vi "Set multiple channels.vi"(6 "timeout (ms)":i32, 8 "values":dbl[](array[numeric]), 9 "names":string[](array[string]), 10 "Gateway IP Address (\"\": localhost)":string, 11 "Sequence Context":refnum<k7>) -> (0 "error out":errorcluster, 1 "timed out?":bool, 2 "Report Text":string)   [LabVIEW 2014, in "Set Channels.lvlib"]
uses:
  Set Channels.lvlib
  <vilib>/NI Veristand/Execution/Workspace/NI VeriStand - Set Multiple Channel Values.vi
  <vilib>/NI Veristand/Execution/Workspace/NI VeriStand - Get Multiple Channel Values.vi
  <vilib>/NI Veristand/Execution/Workspace/NI_VS Workspace ExecutionAPI.lvlib
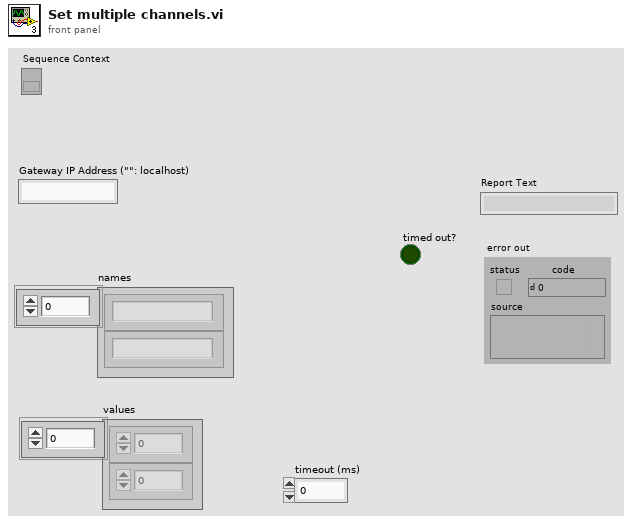
[diagram p1: front panel]
types:
  T1 = typedef "NI_VS Workspace ExecutionAPI.lvlib/WorkspaceAPI.ctl" = refnum<k24>
  T2 = typedef "TestStand - Status Monitor.ctl" = cluster{"Sequence Context":refnum<k7>, "Execution":refnum<k7>, "Termination Monitor":refnum<k7>}
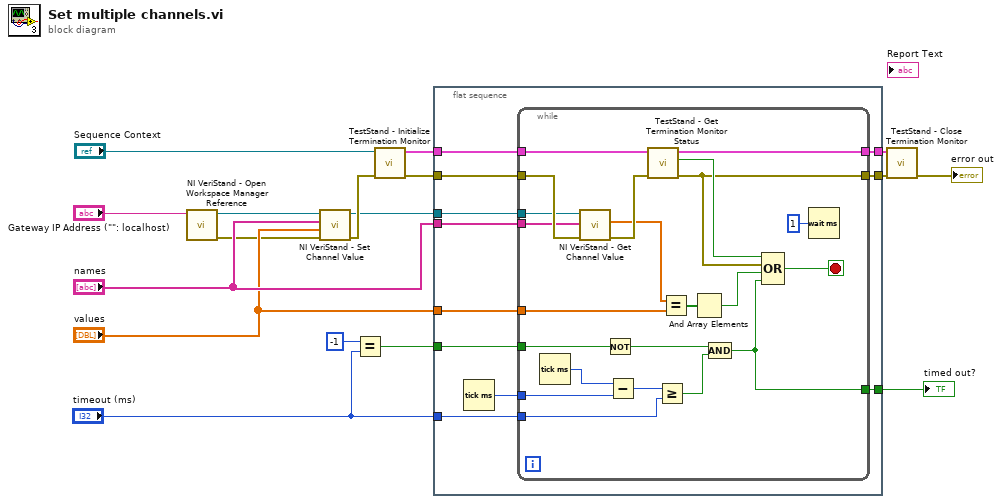
[diagram p0: block diagram]
diagram:
  n1 = call <vilib>:"NI VeriStand - Open Workspace Manager Reference.vi"("Gateway IP Address (\"\": localhost)"="Gateway IP Address (\"\": localhost)") -> ("error out"=w6:errorcluster, "WorkspaceManager"=w7:T1)  [unwired: 9 in]
  n2 = call-poly <vilib>:"NI VeriStand - Set Channel Value.vi"("error in (no error)"=w6, "Values"="values", "Channels"="names", "WorkspaceManager in"=w7) -> ("error out"=w17:errorcluster, "WorkspaceManager out"=w10:T1)  [unwired: 6 in]
  n3 = Equal?(x=-1, y="timeout (ms)") -> (x = y?=w3:bool)
  n4 = call <vilib>:"TestStand - Initialize Termination Monitor.vi"("error in (no error)"=w17, "Sequence Context In"="Sequence Context") -> ("error out"=w11:errorcluster, "Status Monitor Out"=w14:T2)  [unwired: 8 in]
  n5 = flat-sequence {
    tunnel: w14 -> [w28]
    tunnel: [w27] -> w13
    tunnel: [w26] -> w12
    tunnel: w11 -> [w25]
    tunnel: w10 -> [w24]
    tunnel: "names" -> [w23]
    tunnel: "values" -> [w22]
    tunnel: w3 -> [w20]
    tunnel: "timeout (ms)" -> [w19]
    tunnel: [w18] -> w1
    frame #0 {
      n6 = Tick Count (ms)() -> (millisecond timer value=w21:u32)
      n7 = while {
        tunnel: w28 -> [w46]
        tunnel: [w45] -> w27
        tunnel: [w44] -> w26
        tunnel: w25 -> [w42]
        tunnel: w24 -> [w41]
        tunnel: w23 -> [w40]
        tunnel: w22 -> [w39]
        tunnel: w21 -> [w36]
        tunnel: w20 -> [w30]
        tunnel: w19 -> [w32]
        tunnel: [w31] -> w18
        stop <- w43 stop-if-true
        n8 = Tick Count (ms)() -> (millisecond timer value=w35:u32)
        n9 = call-poly <vilib>:"NI VeriStand - Get Channel Value.vi"("error in (no error)"=w42, "Channels"=w40, "WorkspaceManager in"=w41) -> ("error out"=w50:errorcluster, "Values"=w49:dbl[])  [unwired: 6 in, 1 out]
        n10 = Not(x=w30) -> (.not. x?=w29:bool)
        n11 = Subtract(x=w35, y=w36) -> (x-y=w34:u32)
        n12 = call <vilib>:"TestStand - Get Termination Monitor Status.vi"("error in (no error)"=w50, "Status Monitor In"=w46) -> ("error out"=w44:errorcluster, "Terminating or Aborting"=w48:bool, "Status Monitor Out"=w45:T2)  [unwired: 7 in]
        n13 = Greater Or Equal?(x=w34, y=w32) -> (x >= y?=w33:bool)
        n14 = Equal?(x=w49, y=w39) -> (x = y?=w38:bool[])
        n15 = And Array Elements(Boolean array=w38) -> (logical AND=w37:bool)
        n16 = Compound Arithmetic op=AND(w29, w33) -> (w31:bool)
        n17 = Compound Arithmetic op=OR(w48, w44, w37, w31) -> (w43:bool)
        n18 = Wait (ms)(milliseconds to wait=u32 1) -> ()  [unwired: 1 out]
      }
    }
  }
  n19 = call <vilib>:"TestStand - Close Termination Monitor.vi"("error in (no error)"=w12, "Status Monitor In"=w13) -> ("error out"=→"error out":errorcluster)  [unwired: 9 in]
  "timed out?" <- w1
